vi "Get Frame Info From XNET Cluster.vi"(8 "error in (no error)":errorcluster, 11 "Cluster In":refnum<k21>) -> (0 "error out":errorcluster, 1 "Frame IDs":u32[](array[numeric]), 2 "Frame Names":string[](array[string]), 3 "Frame Info":T1[](array[typedef]))   [LabVIEW 2025, in "Protection and Counter Addon System Explorer.lvlib"]
uses:
  Protection and Counter Addon System Explorer.lvlib
  Types/Base Frame Info_NoVS.ctl
  Types/Signal Attributes.ctl
  Types/CAN Filter Type.ctl
  <vilib>/xnet/xnet.llb/XNET Get DBC Mode.ctl
  <vilib>/xnet/xnet.llb/XNET Database Get DBC Attribute (Signal).vi
  <resource>/objmgr/xnet.rc
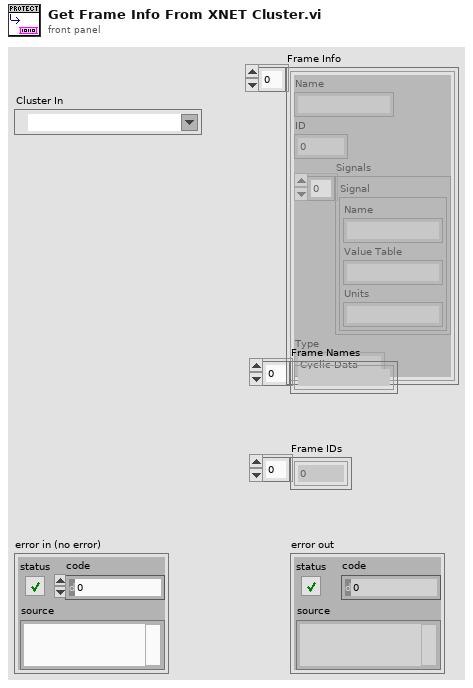
[diagram p1: front panel]
types:
  T1 = typedef "Protection and Counter Addon System Explorer.lvlib/Base Frame Info_NoVS.ctl" = cluster{"Name":string, "ID":u32, "Signals":T2[], "Type":T3}
  T2 = typedef "Protection and Counter Addon System Explorer.lvlib/Signal Attributes.ctl" = cluster{"Name":string, "Value Table":string, "Units":string}
  T3 = typedef "Protection and Counter Addon System Explorer.lvlib/CAN Filter Type.ctl" = enum16{"Cyclic Data", "Event Data", "Cyclic/Event", "All"}
  T4 = typedef "XNET Get DBC Mode.ctl" = u32
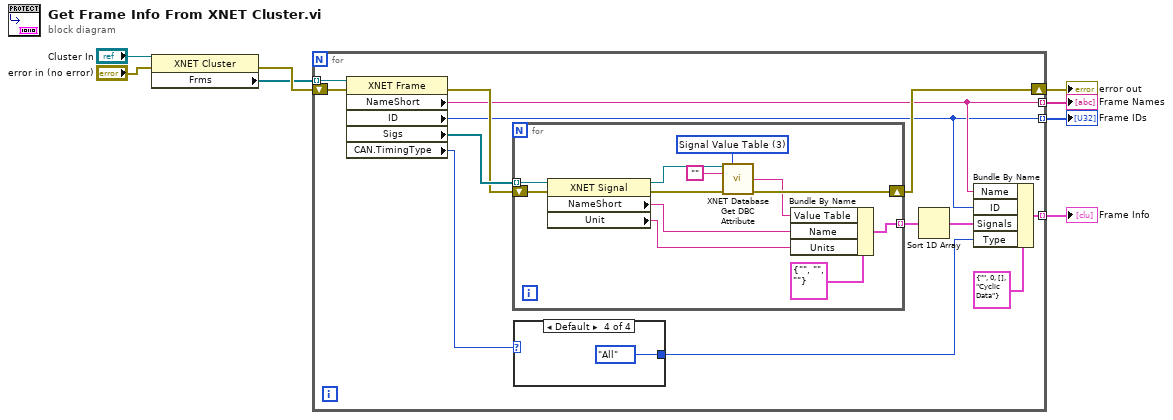
[diagram p0: block diagram]
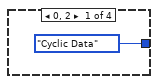
[diagram p2: hidden frame]
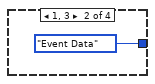
[diagram p3: hidden frame]
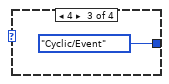
[diagram p4: hidden frame]
diagram:
  n1 = property class="XNET Cluster"(reference="Cluster In", error in="error in (no error)") -> (error out=w2:errorcluster, "Frms"=w1:refnum<k21>[])  [unwired: 1 out]
  n2 = for {
    tunnel: w1 -> [w21] mode=indexing
    shift-right: [w13] -> w5
    shift-left: w2 -> [w20]
    tunnel: [w17] -> w8 mode=indexing
    tunnel: [w12] -> w6 mode=indexing
    tunnel: [w11] -> w7 mode=indexing
    n3 = property class="XNET Frame"(reference=w21, error in=w20) -> (error out=w14:errorcluster, "NameShort"=w12:string, "ID"=w11:u32, "Sigs"=w19:refnum<k21>[], "CAN.TimingType"=w10:u32)  [unwired: 1 out]
    n4 = for {
      tunnel: w19 -> [w37] mode=indexing
      shift-right: [w34] -> w13
      shift-left: w14 -> [w36]
      tunnel: [w30] -> w18 mode=indexing
      w32 = T4 3 items=["Attribute Value", "Enumeration", "Attribute Name List", "Signal Value Table"] ("mode")
      n5 = property class="XNET Signal"(reference=w37, error in=w36) -> (reference out=w33:refnum<k21>, error out=w35:errorcluster, "NameShort"=w31:string, "Unit"=w26:string)
      n6 = call-poly <vilib>:"XNET Database Get DBC Attribute.vi"("signal in"=w33, "mode"=w32, "attribute name"="", "error in (no error)"=w35) -> ("attribute text"=w27:string, "error out"=w34:errorcluster)  [unwired: 8 in, 2 out]
      n7 = Bundle By Name(cluster=T2 {"Name"="", "Value Table"="", "Units"=""}, "Value Table"=w27, "Name"=w31, "Units"=w26) -> (w30:T2)
    }
    n8 = case shown="Default" w10 {
      tunnel: [CAN_Filter_Type."Cyclic Data" ("Type") CAN_Filter_Type."Event Data" ("Type") CAN_Filter_Type."Cyclic/Event" ("Type") CAN_Filter_Type."All" ("Type")] -> w9
      frame 0, 2 {
      }
      frame 1, 3 {
      }
      frame 4 {
      }
      frame Default {
      }
    }
    n9 = Sort 1D Array(array=w18) -> (sorted array=w15:T2[])
    n10 = Bundle By Name(cluster=T1 {"Name"="", "ID"=0, "Signals"=[], "Type"=enum."Cyclic Data"}, "Name"=w12, "ID"=w11, "Signals"=w15, "Type"=w9) -> (w17:T1)
  }
  "Frame Info" <- w8
  "Frame IDs" <- w7
  "Frame Names" <- w6
  "error out" <- w5
